vi "Facade.vi"(0 "Data In":T5, 2 "Display State In":T3, 3 "Container State":T4) -> (6 "Data Out":T5, 7 "Display State Out":T3, 8 "Action":T2)   [LabVIEW 2015, in "Filter.xctl"]
uses:
  Filter.xctl
  Data.vi
  Classes/Filter/Filter.lvclass
  <vilib>/_xctls/Container State.ctl
  State.vi
  <vilib>/_xctls/Action.ctl
  Classes/Filter/Filter.lvclass/Filter.ctl
  Classes/Filter/Shape.ctl
  Classes/Filter/Class.ctl
  Classes/Filter/Read Type.vi
  Classes/Filter/Read Class.vi
  Classes/Filter/Read Order.vi
  Classes/Filter/Read Cascade.vi
  Classes/Filter/Read Units.vi
  Classes/Filter/Read CF (kHz).vi
  Classes/Filter/Read BW (kHz).vi
  Classes/Filter/Write Cascade.vi
  Classes/Filter/Write Class.vi
  Classes/Filter/Write CF (kHz).vi
  Classes/Filter/Write BW (kHz).vi
  Classes/Filter/Write Units.vi
  Classes/Filter/Write Type.vi
  Classes/Filter/Write Order.vi
  <vilib>/_xctls/XControlSupport.lvlib
panel:
  in  "Order":i32
  in  "Class":enum16{"Elliptic", "Butterworth", "Brickwall"}(ring)
  in  "BWUnits":enum16{"kHz", "Octaves", "Min-Max"}(ring) caption="Filter"
  in  "Cascade":bool
  in  "F2":dbl caption="BW"
  in  "Type":T1(ring) caption="Shape"
  in  "F1":dbl caption="CF (kHz)"
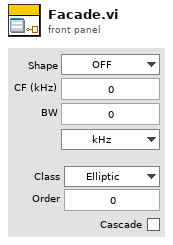
[diagram p1: front panel]
types:
  T1 = enum16{"OFF", "Lowpass", "Highpass", "Bandpass", "Bandstop"}
  T2 = typedef "XControlSupport.lvlib/Action.ctl" = cluster{"Data Changed?":bool, "State Changed?":bool, "Action Name":string}
  T3 = typedef "Filter.xctl/State.vi" = cluster{"Numeric":dbl}
  T4 = typedef "XControlSupport.lvlib/Container State.ctl" = cluster{"Indicator?":bool, "Run Mode?":bool, " Refnum":refnum<vi>}
  T5 = typedef "Filter.xctl/Data.vi" = refnum<class "Filter.lvclass">
  T6 = typedef "Filter.lvclass/Class.ctl" = enum16{"Elliptic", "Butterworth", "Brickwall"}
  T7 = typedef "Filter.lvclass/Shape.ctl" = enum16{"OFF", "Lowpass", "Highpass", "Bandpass", "Bandstop"}
  T8 = typedef "Filter.lvclass/Units.ctl" = enum16{"Linear", "Octaves", "Min-Max"}
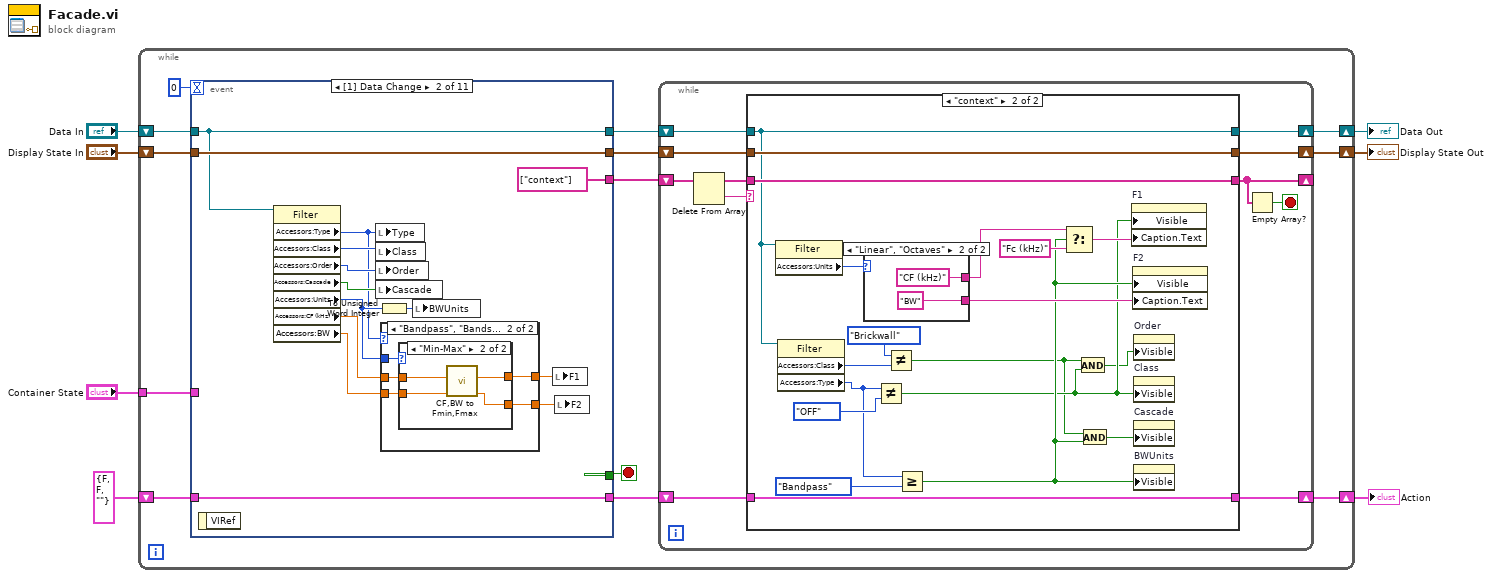
[diagram p0: block diagram]
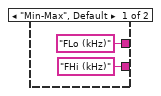
[diagram p3: hidden frame]
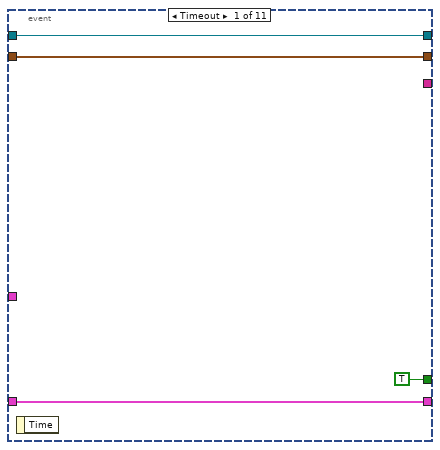
[diagram p4: hidden frame]
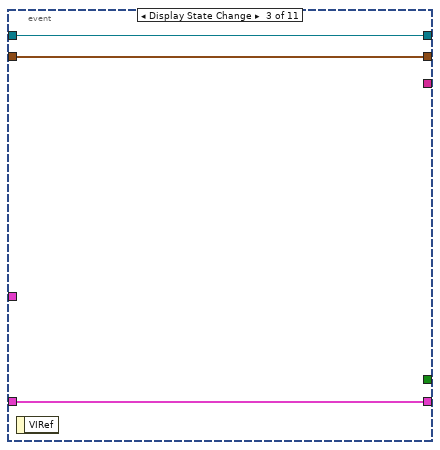
[diagram p7: hidden frame]
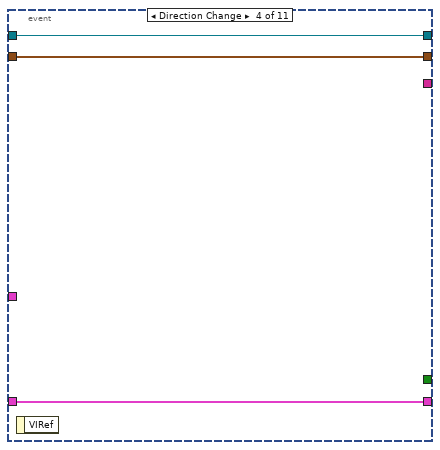
[diagram p8: hidden frame]
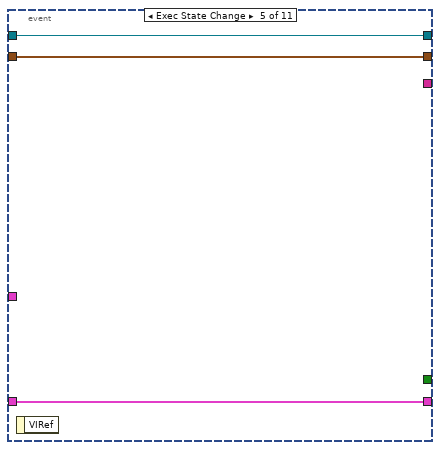
[diagram p9: hidden frame]
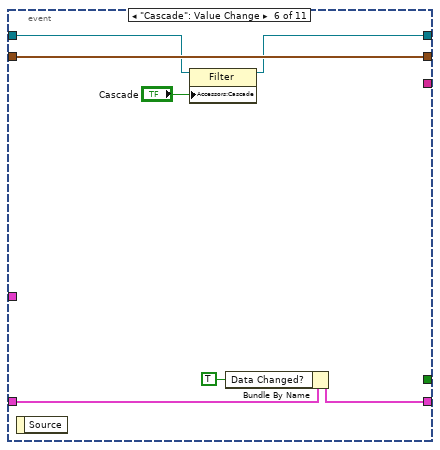
[diagram p10: hidden frame]
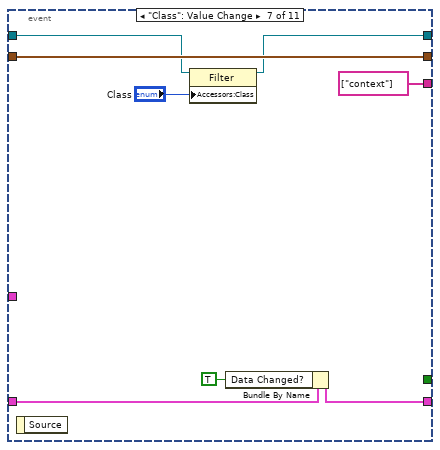
[diagram p11: hidden frame]
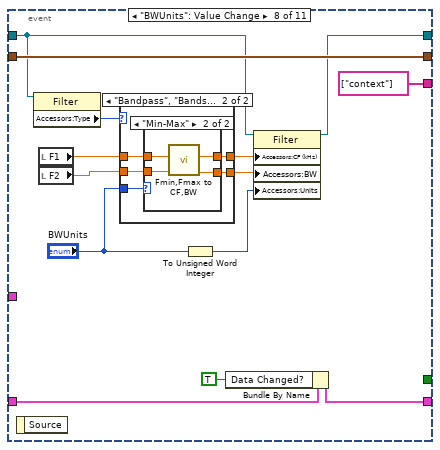
[diagram p12: hidden frame]
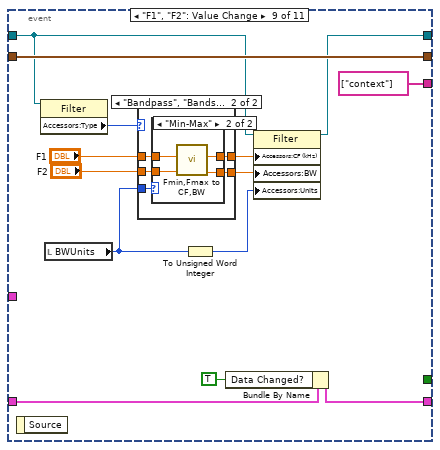
[diagram p15: hidden frame]
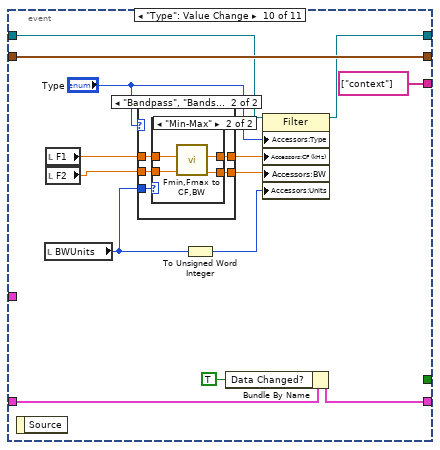
[diagram p18: hidden frame]
diagram:
  n1 = while {
    shift-right: [w11] -> w4
    shift-left: "Display State In" -> [w20]
    tunnel: "Container State" -> [w17]
    shift-right: [w13] -> w7
    shift-left: "Data In" -> [w16]
    shift-right: [w8] -> w2
    shift-left: T2 {"Data Changed?"=FALSE, "State Changed?"=FALSE, "Action Name"=""} ("Action") -> [w15]
    stop <- w19 stop-if-true
    n2 = event shown="[1] Data Change" {
      selector: _ -> [_ _ _ _ _ _ _ _ _ _ _]
      dyn-events: _ -> [_ _ _ _ _ _ _ _ _ _ _]
      timeout: 0 -> [_ _ _ _ _ _ _ _ _ _ _]
      tunnel: w20 -> [w60 w76 w92 w95 w98 w105 w113 w127 w154 w181 w201]
      tunnel: [w60 w76 w92 w95 w98 w105 w113 w127 w154 w181 w201] -> w12
      tunnel: [TRUE _ _ _ _ _ _ _ _ _ _] -> w19
      tunnel: w17 -> [_ _ _ _ _ _ _ _ _ _ _]
      tunnel: w16 -> [w59 w74 w91 w94 w97 w104 w112 w115 w142 w172 w200]
      tunnel: [w59 w74 w91 w94 w97 w102 w109 w124 w151 w178 w198] -> w14
      tunnel: [w61 w75 w90 w93 w96 w101 w108 w123 w150 w177 w197] -> w9
      tunnel: w15 -> [w61 w75 w90 w93 w96 w103 w111 w126 w153 w180 w199]
      tunnel: [_ string[] ["context"] _ _ _ _ string[] ["context"] string[] ["context"] string[] ["context"] string[] ["context"] _] -> w10
      event Timeout {
        n3 = event-data() -> ()  [unwired: 1 in, 1 out]
      }
      event Data Change {
        n4 = event-data() -> ()  [unwired: 1 in, 1 out]
        n5 = property class="Filter"(reference=w74) -> ("Accessors:Type"=w63:T7, "Accessors:Class"=w73:T6, "Accessors:Order"=w72:i32, "Accessors:Cascade"=w71:bool, "Accessors:Units"=w68:T8, "Accessors:CF (kHz)"=w70:dbl, "Accessors:BW"=w69:dbl)  [unwired: 1 in, 2 out]
        n6 = local write "Type"(w63) -> ()
        n7 = local write "Class"(w73) -> ()
        n8 = local write "Order"(w72) -> ()
        n9 = local write "Cascade"(w71) -> ()
        n10 = To Unsigned Word Integer(number=w68) -> (unsigned 16bit integer=w64:u16)
        n11 = case shown="\"Bandpass\", \"Bandstop\"" w63 {
          tunnel: w70 -> [w78 w83]
          tunnel: w69 -> [w77 w82]
          tunnel: w68 -> [_ w81]
          tunnel: [w78 w80] -> w67
          tunnel: [w77 w79] -> w66
          frame "OFF", Default {
          }
          frame "Bandpass", "Bandstop" {
            n12 = case shown="\"Min-Max\"" w81 {
              tunnel: [w85 w87] -> w80
              tunnel: [w84 w86] -> w79
              tunnel: w83 -> [w85 w89]
              tunnel: w82 -> [w84 w88]
              frame "Linear", Default {
              }
              frame "Min-Max" {
                n13 = call "CF,BW to Fmin,Fmax.vi"("BW"=w88, "CF"=w89) -> ("Fmax"=w86:dbl, "Fmin"=w87:dbl)  [unwired: 8 in]
              }
            }
          }
        }
        n14 = local write "BWUnits"(w64) -> ()
        n15 = local write "F1"(w67) -> ()
        n16 = local write "F2"(w66) -> ()
      }
      event Display State Change {
        n17 = event-data() -> ()  [unwired: 1 in, 1 out]
      }
      event Direction Change {
        n18 = event-data() -> ()  [unwired: 1 in, 1 out]
      }
      event Exec State Change {
        n19 = event-data() -> ()  [unwired: 1 in, 1 out]
      }
      event "Cascade": Value Change {
        n20 = event-data() -> ()  [unwired: 1 in, 1 out]
        n21 = property class="Filter"(reference=w104, "Accessors:Cascade"="Cascade") -> (reference out=w102:T5)  [unwired: 1 in, 1 out]
        n22 = Bundle By Name(cluster=w103, "Data Changed?"=TRUE) -> (w101:T2)
      }
      event "Class": Value Change {
        n23 = event-data() -> ()  [unwired: 1 in, 1 out]
        n24 = property class="Filter"(reference=w112, "Accessors:Class"="Class") -> (reference out=w109:T5)  [unwired: 1 in, 1 out]
        n25 = Bundle By Name(cluster=w111, "Data Changed?"=TRUE) -> (w108:T2)
      }
      event "BWUnits": Value Change {
        n26 = event-data() -> ()  [unwired: 1 in, 1 out]
        n27 = property class="Filter"(reference=w115) -> ("Accessors:Type"=w114:T7)  [unwired: 1 in, 2 out]
        n28 = local read "F1"() -> (w119:dbl)
        n29 = local read "F2"() -> (w118:dbl)
        n30 = case shown="\"Bandpass\", \"Bandstop\"" w114 {
          tunnel: [w129 w134] -> w121
          tunnel: [w128 w133] -> w120
          tunnel: w119 -> [w129 w132]
          tunnel: w118 -> [w128 w131]
          tunnel: "BWUnits" -> [_ w130]
          frame "OFF", Default {
          }
          frame "Bandpass", "Bandstop" {
            n31 = case shown="\"Min-Max\"" w130 {
              tunnel: [w136 w140] -> w134
              tunnel: [w135 w139] -> w133
              tunnel: w132 -> [w136 w138]
              tunnel: w131 -> [w135 w137]
              frame "kHz", Default {
              }
              frame "Min-Max" {
                n32 = call "Fmin,Fmax to CF,BW.vi"("Fmax"=w137, "Fmin"=w138) -> ("BW"=w139:dbl, "CF"=w140:dbl)  [unwired: 8 in]
              }
            }
          }
        }
        n33 = To Unsigned Word Integer(number="BWUnits") -> (unsigned 16bit integer=w116:u16)
        n34 = Bundle By Name(cluster=w126, "Data Changed?"=TRUE) -> (w123:T2)
        n35 = property class="Filter"(reference=w115, "Accessors:CF (kHz)"=w121, "Accessors:BW"=w120, "Accessors:Units"=w116) -> (reference out=w124:T5)  [unwired: 1 in, 1 out]
      }
      event "F1", "F2": Value Change {
        n36 = event-data() -> ()  [unwired: 1 in, 1 out]
        n37 = property class="Filter"(reference=w142) -> ("Accessors:Type"=w141:T7)  [unwired: 1 in, 2 out]
        n38 = local read "BWUnits"() -> (w145:enum16{"kHz", "Octaves", "Min-Max"})
        n39 = case shown="\"Bandpass\", \"Bandstop\"" w141 {
          tunnel: [w156 w161] -> w148
          tunnel: [w155 w160] -> w147
          tunnel: w145 -> [_ w159]
          tunnel: "F1" -> [w156 w158]
          tunnel: "F2" -> [w155 w157]
          frame "OFF", Default {
          }
          frame "Bandpass", "Bandstop" {
            n40 = case shown="\"Min-Max\"" w159 {
              tunnel: [w163 w167] -> w161
              tunnel: [w162 w166] -> w160
              tunnel: w158 -> [w163 w165]
              tunnel: w157 -> [w162 w164]
              frame "kHz", Default {
              }
              frame "Min-Max" {
                n41 = call "Fmin,Fmax to CF,BW.vi"("Fmax"=w164, "Fmin"=w165) -> ("BW"=w166:dbl, "CF"=w167:dbl)  [unwired: 8 in]
              }
            }
          }
        }
        n42 = To Unsigned Word Integer(number=w145) -> (unsigned 16bit integer=w146:u16)
        n43 = Bundle By Name(cluster=w153, "Data Changed?"=TRUE) -> (w150:T2)
        n44 = property class="Filter"(reference=w142, "Accessors:CF (kHz)"=w148, "Accessors:BW"=w147, "Accessors:Units"=w146) -> (reference out=w151:T5)  [unwired: 1 in, 1 out]
      }
      event "Type": Value Change {
        n45 = event-data() -> ()  [unwired: 1 in, 1 out]
        n46 = local read "BWUnits"() -> (w173:enum16{"kHz", "Octaves", "Min-Max"})
        n47 = local read "F1"() -> (w169:dbl)
        n48 = local read "F2"() -> (w168:dbl)
        n49 = case shown="\"Bandpass\", \"Bandstop\"" "Type" {
          tunnel: [w183 w188] -> w171
          tunnel: [w182 w187] -> w175
          tunnel: w173 -> [_ w186]
          tunnel: w169 -> [w183 w185]
          tunnel: w168 -> [w182 w184]
          frame "OFF", Default {
          }
          frame "Bandpass", "Bandstop" {
            n50 = case shown="\"Min-Max\"" w186 {
              tunnel: [w190 w194] -> w188
              tunnel: [w189 w193] -> w187
              tunnel: w185 -> [w190 w192]
              tunnel: w184 -> [w189 w191]
              frame "kHz", Default {
              }
              frame "Min-Max" {
                n51 = call "Fmin,Fmax to CF,BW.vi"("Fmax"=w191, "Fmin"=w192) -> ("BW"=w193:dbl, "CF"=w194:dbl)  [unwired: 8 in]
              }
            }
          }
        }
        n52 = To Unsigned Word Integer(number=w173) -> (unsigned 16bit integer=w174:u16)
        n53 = Bundle By Name(cluster=w180, "Data Changed?"=TRUE) -> (w177:T2)
        n54 = property class="Filter"(reference=w172, "Accessors:Type"="Type", "Accessors:CF (kHz)"=w171, "Accessors:BW"=w175, "Accessors:Units"=w174) -> (reference out=w178:T5)  [unwired: 1 in, 1 out]
      }
      event "Order": Value Change {
        n55 = event-data() -> ()  [unwired: 1 in, 1 out]
        n56 = property class="Filter"(reference=w200, "Accessors:Order"="Order") -> (reference out=w198:T5)  [unwired: 1 in, 1 out]
        n57 = Bundle By Name(cluster=w199, "Data Changed?"=TRUE) -> (w197:T2)
      }
    }
    n58 = while {
      shift-right: [w28] -> _
      shift-left: w10 -> [w31]
      shift-right: [w23] -> w11
      shift-left: w12 -> [w24]
      shift-right: [w25] -> w13
      shift-left: w14 -> [w26]
      shift-right: [w22] -> w8
      shift-left: w9 -> [w21]
      stop <- w27 stop-if-true
      n59 = Delete From Array(array=w31) -> (deleted portion=w29:string, array with subset deleted=w30:string[])  [unwired: 2 in]
      n60 = case shown="\"context\"" w29 {
        tunnel: w30 -> [w35 w54]
        tunnel: [w35 w54] -> w28
        tunnel: w26 -> [w34 w46]
        tunnel: [w34 w46] -> w25
        tunnel: w24 -> [w33 w53]
        tunnel: [w33 w53] -> w23
        tunnel: [w32 w52] -> w22
        tunnel: w21 -> [w32 w52]
        frame "", Default {
        }
        frame "context" {
          n61 = property class="Filter"(reference=w46) -> ("Accessors:Units"=w51:T8)  [unwired: 1 in, 2 out]
          n62 = property class="Filter"(reference=w46) -> ("Accessors:Class"=w41:T6, "Accessors:Type"=w42:T7)  [unwired: 1 in, 2 out]
          n63 = case shown="\"Linear\", \"Octaves\"" w51 {
            tunnel: ["FLo (kHz)" "CF (kHz)"] -> w47
            tunnel: ["FHi (kHz)" "BW"] -> w48
            frame "Min-Max", Default {
            }
            frame "Linear", "Octaves" {
            }
          }
          n64 = Not Equal?(x=w42, y=Shape."OFF") -> (x != y?=w39:bool)
          n65 = Not Equal?(x=Class."Brickwall", y=w41) -> (x != y?=w36:bool)
          n66 = Greater Or Equal?(x=w42, y=Shape."Bandpass") -> (x >= y?=w44:bool)
          n67 = Select(t=w47, s=w44, f="Fc (kHz)" ("t")) -> (s? t:f=w49:string)
          n68 = And(x=w36, y=w39) -> (x .and. y?=w38:bool)
          n69 = And(x=w36, y=w44) -> (x .and. y?=w37:bool)
          n70 = property on="F1" class="DigNum (strict)"("Visible"=w39, "Caption.Text"=w49) -> ()  [unwired: 2 in, 2 out]
          n71 = property on="F2" class="DigNum (strict)"("Visible"=w44, "Caption.Text"=w48) -> ()  [unwired: 2 in, 2 out]
          n72 = property on="Order" class="DigNum (strict)"("Visible"=w38) -> ()  [unwired: 2 in, 2 out]
          n73 = property on="Class" class="Enum (strict)"("Visible"=w39) -> ()  [unwired: 2 in, 2 out]
          n74 = property on="Cascade" class="Bool (strict)"("Visible"=w37) -> ()  [unwired: 2 in, 2 out]
          n75 = property on="BWUnits" class="Enum (strict)"("Visible"=w44) -> ()  [unwired: 2 in, 2 out]
        }
      }
      n76 = Empty Array?(array=w28) -> (empty?=w27:bool)
    }
  }
  "Display State Out" <- w4
  "Data Out" <- w7
  "Action" <- w2
